vi "Mailbox.vi"(8 "error in (no error)":errorcluster) -> (0 "error out":errorcluster, 3 "System Status Actor":refnum<event-registration>)   [LabVIEW 2020, in "System Status Actor API.lvclass"]
uses:
  System Status Actor API.lvclass
  Actor/Status.ctl
  <vilib>/Utility/RT CPU Load.ctl
  C:/dev/PGS/2001 - TBCM/Source/RT/RTAF/Source/RTAF/Actors/Base Actor/API/Actor API.lvclass
  RTAF Global References.vi
  Base Actor/API/Actor API.lvclass
  <vilib>/NI_Real-Time Target Support.lvlib
  Actor/System Status Actor.lvclass
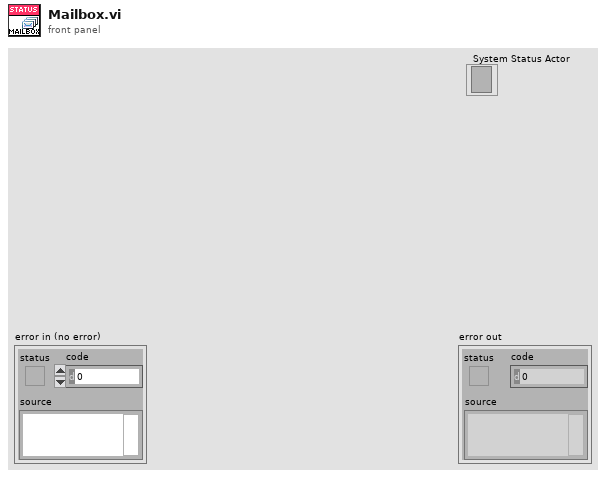
[diagram p1: front panel]
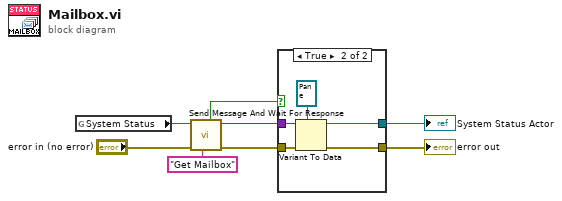
[diagram p0: block diagram]
diagram:
  n1 = global read "RTAF Global References.vi" "System Status"() -> (w6:refnum<class "System Status Actor API.lvclass">)
  n2 = call "Send Message And Wait For Response.vi"("Name"="Get Mailbox", "error in (no error)"="error in (no error)", "Actor API in"=w6) -> ("error out"=w4:errorcluster, "Response"=w3:variant, "Response Received"=w5:bool)  [unwired: 6 in]
  n3 = case shown="True" w5 {
    tunnel: w4 -> [w9 w14]
    tunnel: w3 -> [_ w13]
    tunnel: [_ w11] -> w1
    tunnel: [w9 w10] -> w2
    frame False {
    }
    frame True {
      n4 = Variant To Data(error in=w14, type=refnum<event-registration> refnum ("System Status Actor"), Variant=w13) -> (data=w11:refnum<event-registration>, error out=w10:errorcluster)
    }
  }
  "error out" <- w2
  "System Status Actor" <- w1
